vi "Get SLSC Switch Properties.vi"(8 "error in (no error)":errorcluster, 9 "Number of Paired Channels":i32=4, 10 "Number of DUT-Load Channels":i32=8, 11 "device":refnum<k21>="SLSC-12001-0317E1AA-Mod2") -> (0 "error out":errorcluster, 2 "SLSC Switch States":T1)   [LabVIEW 2020, in "SLSC Switch System Tests.lvclass"]
uses:
  SLSC Switch System Tests.lvclass
  SLSC Switch States.ctl
  <vilib>/SLSC/Initialize Session with Devices.vi
  <vilib>/SLSC/Get Phys Chan Property (I32).vi
  <vilib>/SLSC/Close Session.vi
  <vilib>/SLSC/SLSC.lvlib
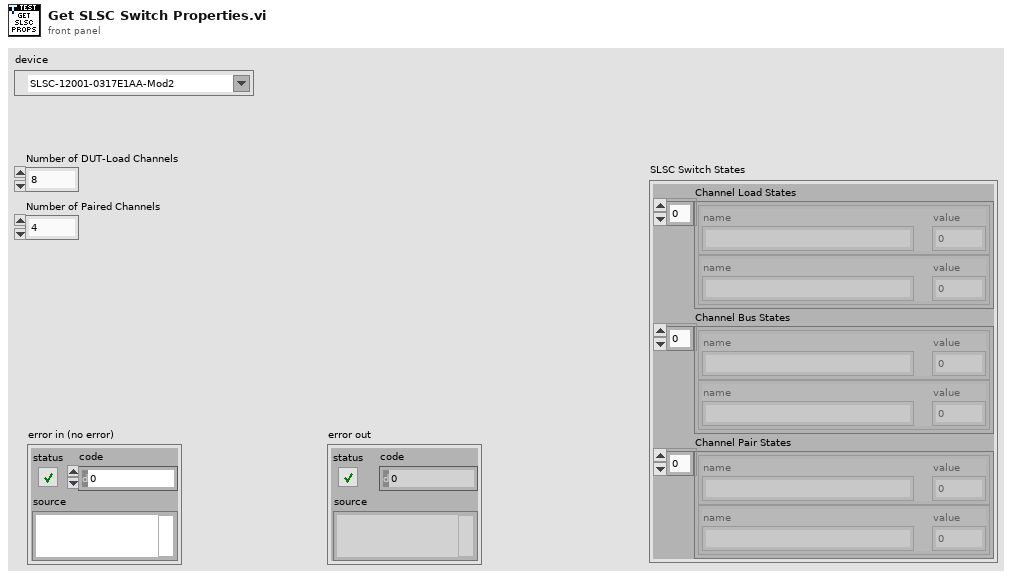
[diagram p1: front panel]
types:
  T1 = typedef "SLSC Switch System Tests.lvclass/SLSC Switch States.ctl" = cluster{"Channel Load States":cluster{"name":string, "value":i32}[], "Channel Bus States":cluster{"name":string, "value":i32}[], "Channel Pair States":cluster{"name":string, "value":i32}[]}
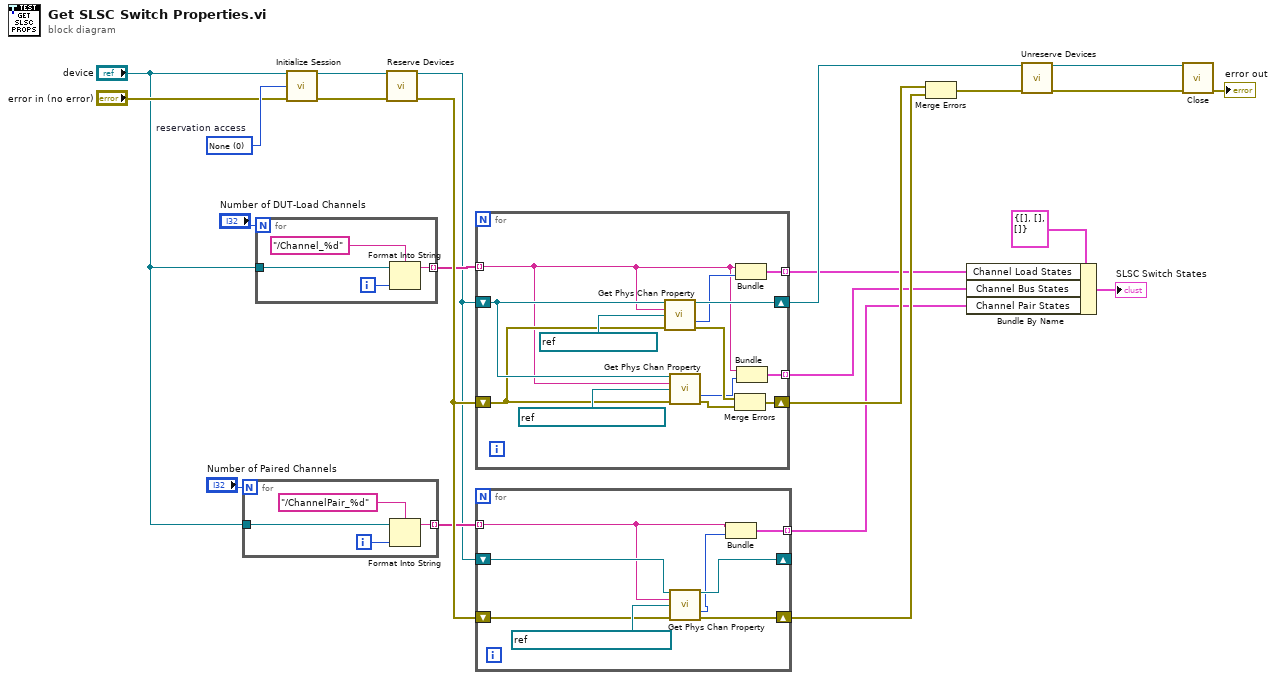
[diagram p0: block diagram]
diagram:
  w23 = 0 items=["None"=0, "Read Only"=1, "Read/Write"=3]  # reservation access
  n1 = for {
    N: "Number of Paired Channels" -> [_]
    tunnel: "device" -> [w26]
    tunnel: [w25] -> w11 mode=indexing
    i -> [w24]
    n2 = Format Into String(format string="/ChannelPair_%d", initial string=w26, w24) -> (resulting string=w25:string)  [unwired: 1 in, 1 out]
  }
  n3 = for {
    N: "Number of DUT-Load Channels" -> [_]
    tunnel: "device" -> [w29]
    tunnel: [w30] -> w13 mode=indexing
    i -> [w28]
    n4 = Format Into String(format string="/Channel_%d", initial string=w29, w28) -> (resulting string=w30:string)  [unwired: 1 in, 1 out]
  }
  n5 = call-poly <vilib>:"Initialize Session.vi"("devices"="device", "reservation access (Read/Write)"=w23, "error in (no error)"="error in (no error)") -> ("session out"=w1:refnum<k21>, "error out"=w19:errorcluster)  [unwired: 11 in]
  n6 = call <vilib>:"Reserve Devices.vi"("session in"=w1, "error in (no error)"=w19) -> ("session out"=w2:refnum<k21>, "error out"=w16:errorcluster)  [unwired: 12 in]
  n7 = for {
    tunnel: w13 -> [w34] mode=indexing
    shift-right: [w43] -> w21
    shift-left: w2 -> [w39]
    shift-right: [w41] -> w9
    shift-left: w16 -> [w38]
    tunnel: [w35] -> w7 mode=indexing
    tunnel: [w32] -> w6 mode=indexing
    n8 = call-poly <vilib>:"Get Phys Chan Property.vi"("session in"=w39, "physical channels"=w34, "property"=refnum<k21> "NI.FIU.State.Load", "error in (no error)"=w38) -> ("session out"=w43:refnum<k21>, "property value"=w36:i32, "error out"=w42:errorcluster)  [unwired: 9 in]
    n9 = call-poly <vilib>:"Get Phys Chan Property.vi"("session in"=w39, "physical channels"=w34, "property"=refnum<k21> "NI.FIU.State.BusSource", "error in (no error)"=w38) -> ("property value"=w33:i32, "error out"=w37:errorcluster)  [unwired: 9 in, 1 out]
    n10 = Merge Errors(w42, w37) -> (w41:errorcluster)
    n11 = Bundle(w34, "property value"=w36) -> (w35:cluster{string, "property value":i32})  [unwired: 1 in]
    n12 = Bundle(w34, "property value"=w33) -> (w32:cluster{string, "property value":i32})  [unwired: 1 in]
  }
  n13 = for {
    shift-right: [w48] -> _
    shift-left: w2 -> [w50]
    shift-right: [w49] -> w10
    shift-left: w16 -> [w51]
    tunnel: w11 -> [w47] mode=indexing
    tunnel: [w45] -> w5 mode=indexing
    n14 = call-poly <vilib>:"Get Phys Chan Property.vi"("session in"=w50, "physical channels"=w47, "property"=refnum<k21> "NI.FIU.State.InterChannel", "error in (no error)"=w51) -> ("session out"=w48:refnum<k21>, "property value"=w46:i32, "error out"=w49:errorcluster)  [unwired: 9 in]
    n15 = Bundle(w47, "property value"=w46) -> (w45:cluster{string, "property value":i32})  [unwired: 1 in]
  }
  n16 = Merge Errors(w9, w10) -> (w15:errorcluster)
  n17 = Bundle By Name(cluster=T1 {"Channel Load States"=[], "Channel Bus States"=[], "Channel Pair States"=[]} ("SLSC Switch States"), "Channel Load States"=w7, "Channel Bus States"=w6, "Channel Pair States"=w5) -> (→"SLSC Switch States":T1)
  n18 = call <vilib>:"Unreserve Devices.vi"("session in"=w21, "error in (no error)"=w15) -> ("session out"=w22:refnum<k21>, "error out"=w18:errorcluster)  [unwired: 12 in]
  n19 = call-poly <vilib>:"Close.vi"("session in"=w22, "error in (no error)"=w18) -> ("error out"=→"error out":errorcluster)  [unwired: 13 in]
